vi "CB Arm Model.vi"() -> ()   [LabVIEW 2020]
uses:
  Motors/CB Motor ID.ctl
panel:
  in  "Motor ID":T1
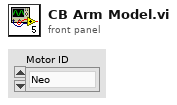
[diagram p1: front panel]
types:
  T1 = typedef "CB Motor ID.ctl" = enum16{"Neo", "Neo 550", "Falcon 500", "775pro"}
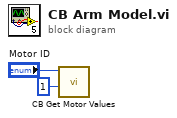
[diagram p0: block diagram]
diagram:
  n1 = call "CB Get Motor Values.vi"("num motors"=1, "Motor ID"="Motor ID") -> ()  [unwired: 6 in, 4 out]
